vi "URI.vi"(11 "IErrorHandler in":refnum<class "ErrorHandler MsgPack.lvclass">) -> (2 "URI":string, 3 "IErrorHandler out":refnum<class "ErrorHandler MsgPack.lvclass">)   [LabVIEW 2020, in "wamplv.lvlib" / "ErrorHandler MsgPack.lvclass"]
uses:
  ErrorHandler MsgPack.lvclass
  ErrorHandler MsgPack.lvclass/ErrorHandler MsgPack.ctl
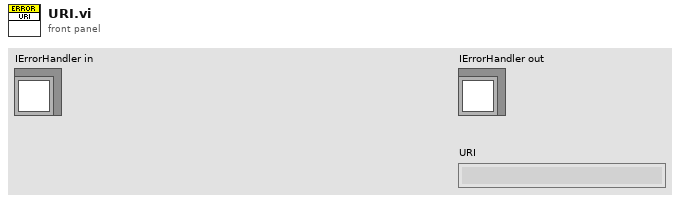
[diagram p1: front panel]
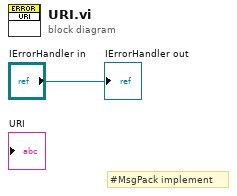
[diagram p0: block diagram]
diagram:
  # "#MsgPack implement"
  "IErrorHandler out" <- "IErrorHandler in"
